vi "testFrequenz.vi"() -> ()   [LabVIEW 2014]
uses:
  <vilib>/DAQmx/read.llb/DAQmx Read (Counter DBL 1Chan 1Samp).vi
  <vilib>/DAQmx/miscellaneous.llb/DAQmx Fill In Error Info.vi
panel:
  out "frequency":dbl caption="Frequenz"
  in  "Stopp":bool
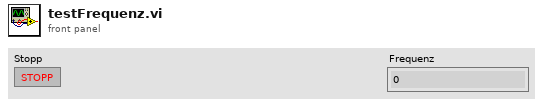
[diagram p1: front panel]
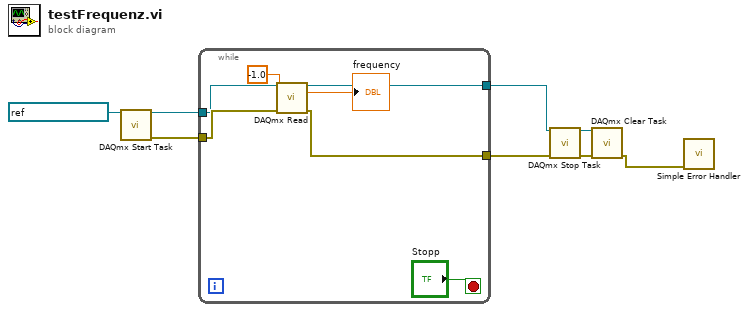
[diagram p0: block diagram]
diagram:
  n1 = call <vilib>:"DAQmx Start Task.vi"("task/channels in"=refnum<k21> "FrequenzTask") -> ("task out"=w7:refnum<k21>, "error out"=w6:errorcluster)  [unwired: 13 in]
  n2 = while {
    tunnel: w7 -> [w12]
    tunnel: w6 -> [w13]
    tunnel: [w14] -> w2
    tunnel: [w11] -> w1
    stop <- "Stopp" stop-if-true
    n3 = call-poly <vilib>:"DAQmx Read.vi"("task/channels in"=w12, "timeout"=-1.0, "error in"=w13) -> ("task out"=w11:refnum<k21>, "data"=→"frequency":dbl, "error out"=w14:errorcluster)  [unwired: 10 in]
  }
  n4 = call <vilib>:"DAQmx Stop Task.vi"("task/channels in"=w1, "error in"=w2) -> ("task out"=w5:refnum<k21>, "error out"=w4:errorcluster)  [unwired: 12 in]
  n5 = call <vilib>:"DAQmx Clear Task.vi"("task in"=w5, "error in"=w4) -> ("error out"=w3:errorcluster)  [unwired: 13 in]
  n6 = call <vilib>:"Simple Error Handler.vi"("error in (no error)"=w3) -> ()  [unwired: 4 in, 5 out]
